vi "XIPIN_LTE_RACH_Detector_1_0.vi"   [LabVIEW 2017]
doc: "LTE Rach decoder.\n------------------------------------\n<b>Need License</b> : Yes"
uses:
  <vilib>/rvi/XilinxIP/XIPIN_XNode/niFpgaXIPIN.xnode
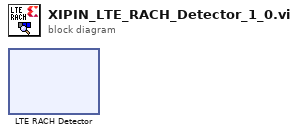
[diagram p0: block diagram]
diagram:
  n1 = xnode ("LTE RACH Detector")() -> ()
